vi "delete img.vi"(8 "error in (no error)":errorcluster caption="Fehler (Eingang, kein Fehler)", 10 "Index":i32, 11 "Segment (Eingang)":refnum<class "Segment.lvclass">) -> (0 "error out":errorcluster caption="Fehler (Ausgang)", 3 "Segment (Ausgang)":refnum<class "Segment.lvclass">)   [LabVIEW 2013, in "DatenKlassen.lvlib" / "Segment.lvclass"]
uses:
  Segment.lvclass
  Segment.lvclass/Segment.ctl
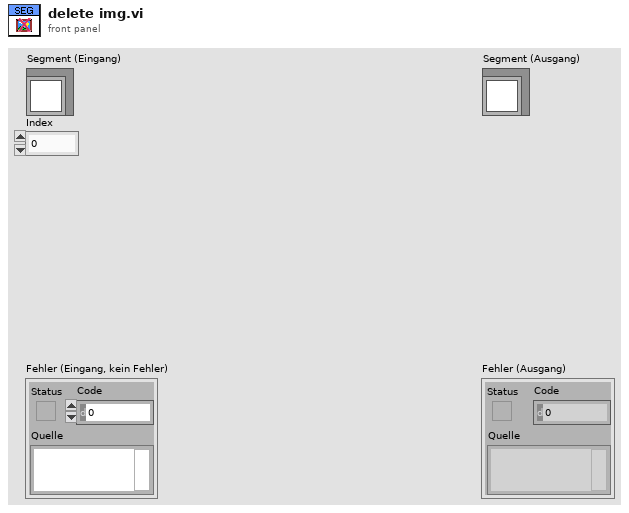
[diagram p1: front panel]
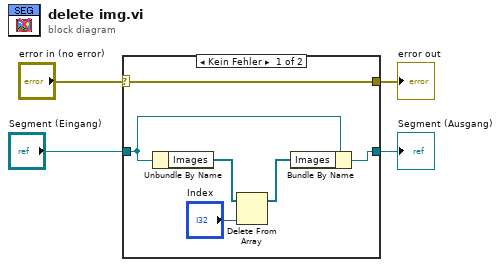
[diagram p0: block diagram]
diagram:
  n1 = case shown="Kein Fehler" "error in (no error)" {
    selector: "error in (no error)" -> [w10 w11]
    tunnel: [w10 w11] -> w3
    tunnel: [w6 w12] -> w1
    tunnel: "Segment (Eingang)" -> [w7 w12]
    frame No Error {
      n2 = Unbundle By Name(w7) -> ("Images"=w9:refnum<class "img.lvclass">[])
      n3 = Delete From Array(array=w9, index="Index") -> (array with subset deleted=w5:refnum<class "img.lvclass">[])  [unwired: 1 in, 1 out]
      n4 = Bundle By Name(cluster=w7, "Images"=w5) -> (w6:refnum<class "Segment.lvclass">)
    }
    frame Error {
    }
  }
  "error out" <- w3
  "Segment (Ausgang)" <- w1
